vi "LMS_DestroyStream.vi"(8 "error in (no error)":errorcluster, 10 "stream":T1, 11 "device_In":i64) -> (0 "error out":errorcluster, 3 "device_Out":i64)   [LabVIEW 2013, in "LMS_LV_Drv.lvlib"]
uses:
  LMS_LV_Drv.lvlib
  Stream_ctl.ctl
  LimeSuite.dll
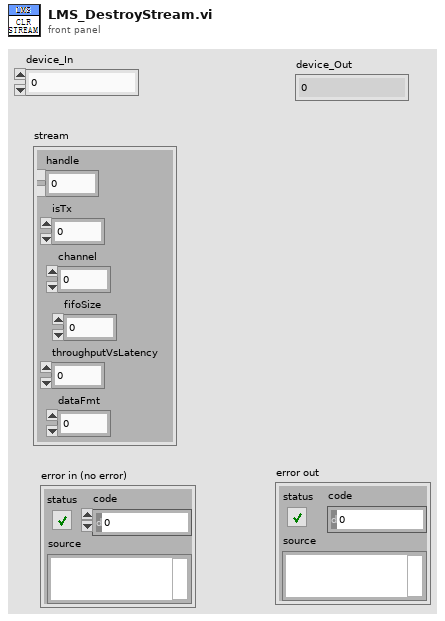
[diagram p1: front panel]
types:
  T1 = typedef "Stream_ctl.ctl" = cluster{"handle":u64, "isTx":u8, "channel":u32, "fifoSize":u32, "throughputVsLatency":dbl, "dataFmt":u32}
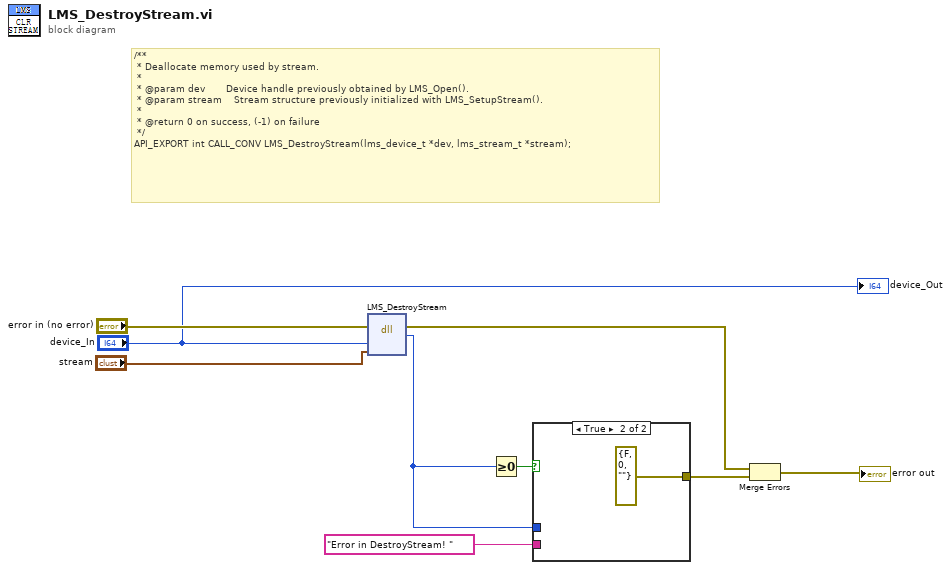
[diagram p0: block diagram]
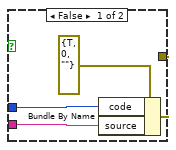
[diagram p2: hidden frame]
diagram:
  # "/**\n * Deallocate memory used by stream.\n *\n * @param dev       Device handle previously obtained by LMS_Open().\n * @param stream    Stream structure previously initialized with LMS_SetupStream().\n *\n * @return 0 on success, (-1) on failure\n */\nAPI_EXPORT int CALL_CONV LMS_DestroyStream(lms_device_t *dev, lms_stream_t *stream);"
  n1 = dll-call lib="D:/SDRDriver/Lab8/LimeSDR_LabVIEW_Driver-master/LimeSuite.dll" fn="LMS_DestroyStream"(error in="error in (no error)", "device"="device_In", "steam"="stream") -> (error out=w2:errorcluster, "return type"=w3:i32)  [unwired: 4 in, 1 out]
  n2 = Greater Or Equal To 0?(x=w3) -> (x >= 0?=w6:bool)
  n3 = case shown="True" w6 {
    tunnel: [w12 errorcluster {"status"=FALSE, "code"=0, "source"=""} ("error in")] -> w4
    tunnel: w3 -> [w11 _]
    tunnel: "Error in DestroyStream! " ("source") -> [w10 _]
    frame False {
      n4 = Bundle By Name(cluster=errorcluster {"status"=TRUE, "code"=0, "source"=""} ("error in"), "code"=w11, "source"=w10) -> (w12:errorcluster)
    }
    frame True {
    }
  }
  n5 = Merge Errors(w2, w4) -> (→"error out":errorcluster)
  "device_Out" <- "device_In"
